vi "B-Field Control Signal Generator.vi"() -> ()   [LabVIEW 2009]
doc: "I. Description:\nThis example demonstrates how to continuously output a waveform using an internal sample clock and a digital start trigger.\n\nII. Instructions for Running:\n1. Select the Physical Channel to correspond to where your signal is output on the DAQ device.\n2. Enter the Minimum and Maximum Voltage Ranges.\n3. Specify the Desired Frequency of the output Waveform\n4. Select the Digital Trigger Source.\n5. Specify the desired Trigger Edge.\n6. Enter the Waveform Information. See the documentation of the Waveform Buffer Generation SubVI for information on each parameter.\n\nIII. Block Diagram Steps:\n1. Create an Analog Output Voltage Task\n2.Call the DAQmx Timing (Use Waveform) VI which sets the sample clock rate based on the input waveform parameters, and set the sample mode to Continuous.\n3. Define the Triggering parameters: Source and Edge\n4. Write the waveform to the output buffer.\n5. Call the Start VI.\n6. Loop continuously until the user presses the Stop button. Check for errors every 100 ms using the Is Task Done? VI\n7. Call the Clear Task VI to clear the Task.\n8. Use the popup dialog box to display an error or warning if any.\n\nIV. I/O Connections Overview:\nMake sure your signal output terminal matches the Physical Channel I/O Control. Also, make sure your digital trigger terminal matches the Trigger Source Control. For further connection information, refer to your hardware reference manual."
uses:
  B-Generator States.ctl
  <vilib>/Utility/error.llb/DialogType.ctl
  <vilib>/DAQmx/write.llb/DAQmx Write (Analog 1D DBL 1Chan NSamp).vi
  <vilib>/DAQmx/configure/trigger.llb/DAQmx Start Trigger (Digital Edge).vi
  <vilib>/DAQmx/configure/timing.llb/DAQmx Timing (Sample Clock).vi
  <vilib>/DAQmx/create/channels.llb/DAQmx Create Channel (AO-Voltage-Basic).vi
  Program Files (x86)/National Instruments/LabVIEW 2009/resource/objmgr/daqmx.rc
panel:
  in  "V5":dbl[unit]=4.0
  in  "V4":dbl[unit]=1.0
  in  "V3":dbl[unit]=-3.0
  in  "V2":dbl[unit]=-5.0
  in  "V1":dbl[unit]=5.0
  in  "D":dbl[unit]=9.999999999999999e-05
  in  "C":dbl[unit]=9.999999999999999e-05
  in  "B":dbl[unit]=9.999999999999999e-05
  in  "A":dbl[unit]=9.999999999999999e-05
  out "B-Field Control Signal":dbl[](graph)
  in  "stop":bool
  # "Example Diagram"
  # "Voltages"
  # "Interval Times"
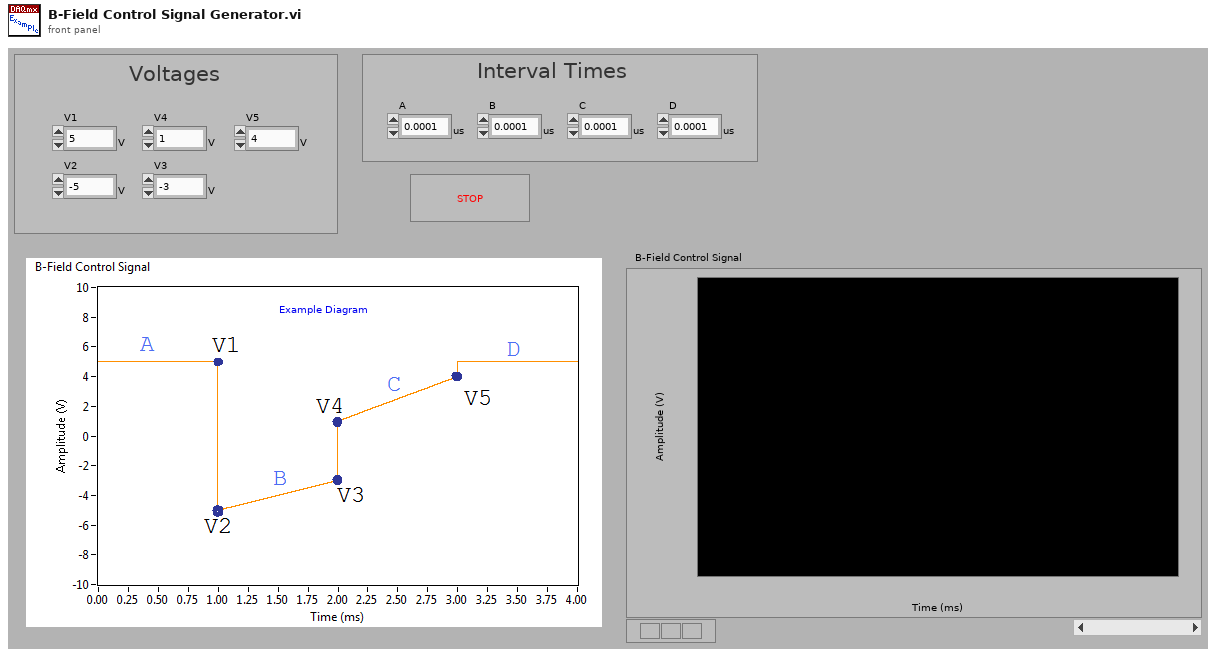
[diagram p1: front panel]
types:
  T1 = typedef "DialogType.ctl" = u16
  T2 = typedef "B-Generator States.ctl" = enum16{"Initialize", "Start Task", "Check Task", "Stop Task", "Stop"}
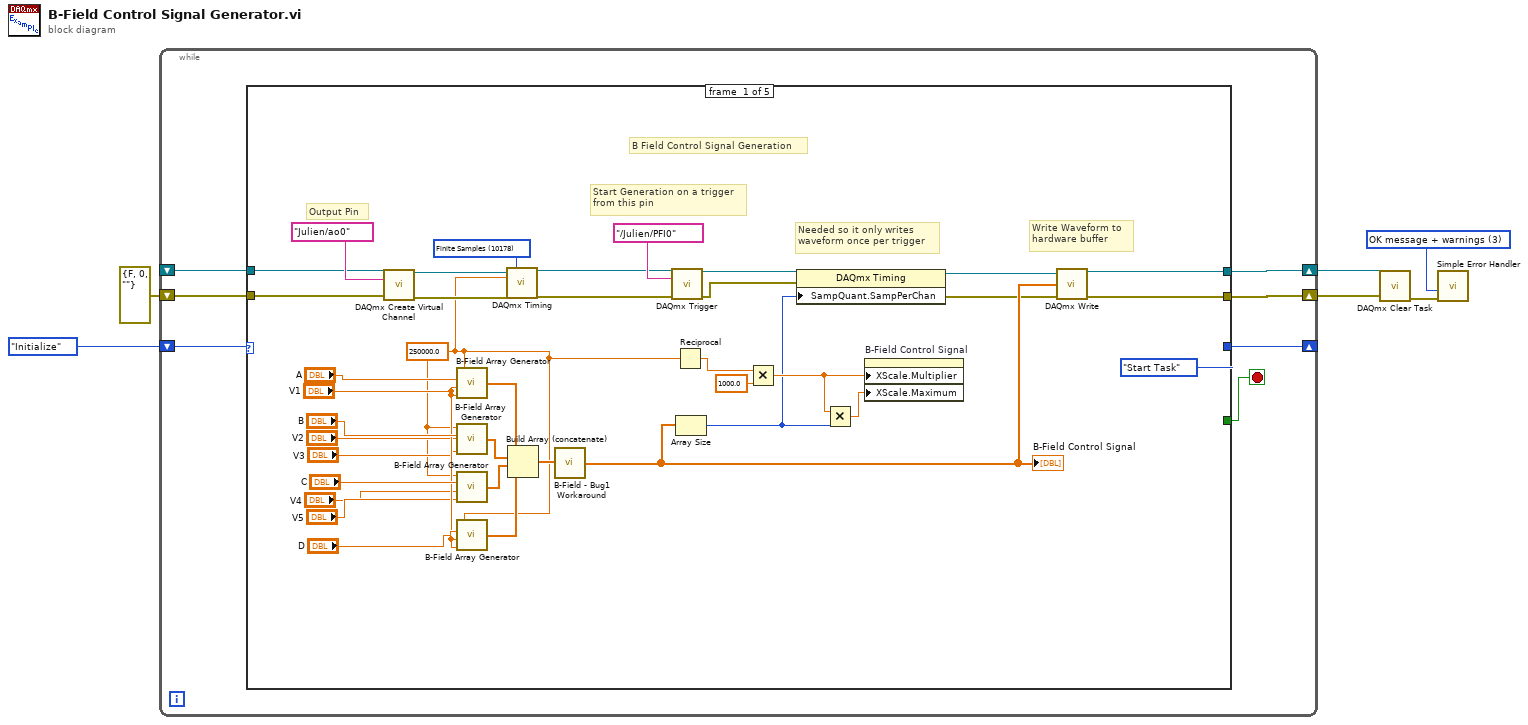
[diagram p0: block diagram]
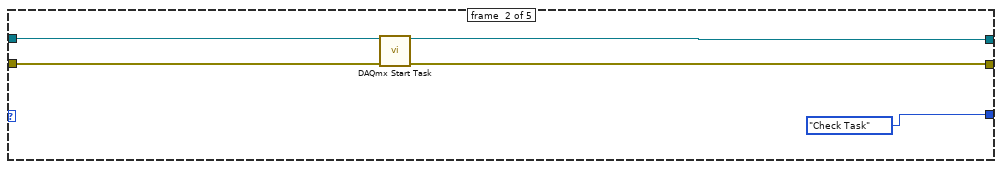
[diagram p2: hidden frame]
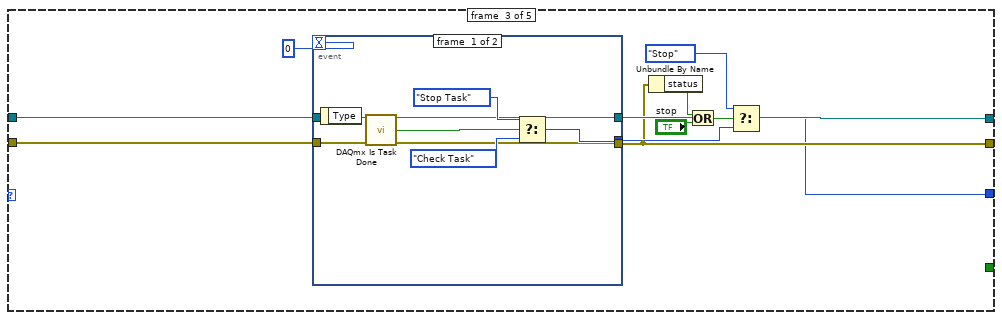
[diagram p3: hidden frame]
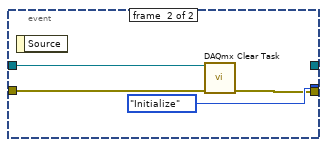
[diagram p4: hidden frame]
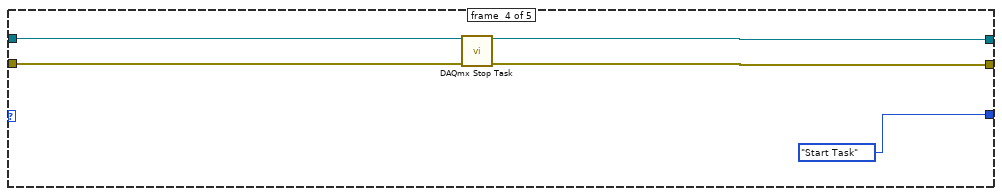
[diagram p5: hidden frame]
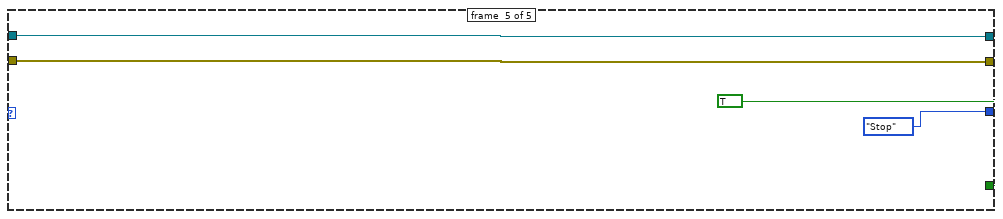
[diagram p6: hidden frame]
diagram:
  w6 = T1 3 items=["no dialog", "OK message", "continue or stop message", "OK message + warnings", "continue/stop + warnings"] ("type of dialog (OK msg:1)")
  n1 = while {
    shift-right: [w10] -> _
    shift-left: B-Generator_States."Initialize" ("B-Generator States") -> [w11]
    shift-right: [w12] -> w3
    shift-left: errorcluster {"status"=FALSE, "code"=0, "source"=""} ("error out") -> [w7]
    shift-right: [w13] -> w4
    shift-left: _ -> [w8]
    stop <- w9 stop-if-true
    n2 = case shown="\"Initialize\"" w11 {
      tunnel: [w29 w52 w58 w81 w85] -> w13
      tunnel: [w28 w53 w57 w80 w84] -> w12
      tunnel: [B-Generator_States."Start Task" ("B-Generator States") B-Generator_States."Check Task" ("B-Generator States") w56 B-Generator_States."Start Task" ("B-Generator States") B-Generator_States."Stop" ("B-Generator States")] -> w10
      tunnel: [_ _ _ _ TRUE] -> w9
      tunnel: w8 -> [w27 w55 w60 w83 w85]
      tunnel: w7 -> [w34 w54 w59 w82 w84]
      frame #0 {
        w23 = 250000.0
        w41 = 10178 items=["Finite Samples"=10178, "Continuous Samples"=10123] ("sample mode")
        # "B Field Control Signal Generation"
        # "Write Waveform to\nhardware buffer"
        # "Output Pin"
        # "Start Generation on a trigger \nfrom this pin"
        # "Needed so it only writes \nwaveform once per trigger"
        n3 = call-poly <vilib>:"DAQmx Create Virtual Channel.vi"("task in"=w27, "physical channels"=tag "Julien/ao0" ("Physical Channels"), "error in"=w34) -> ("task out"=w36:refnum<k21>, "error out"=w35:errorcluster)  [unwired: 7 in, 4 out]
        n4 = call "B-Field Array Generator.vi"("Final Voltage"="V1", "Initial Voltage"="V1", "Time"="A", "Sample Rate"=w23) -> ("Voltage Ouputs"=w33:dbl[])
        n5 = call "B-Field Array Generator.vi"("Final Voltage"="V3", "Initial Voltage"="V2", "Time"="B", "Sample Rate"=w23) -> ("Voltage Ouputs"=w30:dbl[])
        n6 = call "B-Field Array Generator.vi"("Final Voltage"="V5", "Initial Voltage"="V4", "Time"="C", "Sample Rate"=w23) -> ("Voltage Ouputs"=w31:dbl[])
        n7 = call "B-Field Array Generator.vi"("Final Voltage"="V1", "Initial Voltage"="V1", "Time"="D", "Sample Rate"=w23) -> ("Voltage Ouputs"=w32:dbl[])
        n8 = call-poly <vilib>:"DAQmx Timing.vi"("task/channels in"=w36, "sample mode"=w41, "rate"=w23, "error in"=w35) -> ("task out"=w19:refnum<k21>, "error out"=w39:errorcluster)  [unwired: 3 in, 7 out]
        n9 = Build Array (concatenate)(w33, w30, w31, w32) -> (w26:dbl[])
        n10 = call "B-Field - Bug1 Workaround.vi"("Array 2"=w26) -> ("Array"=w24:dbl[])
        "B-Field Control Signal" <- w24
        n11 = call-poly <vilib>:"DAQmx Trigger.vi"("task/channels in"=w19, "source"=tag "/Julien/PFI0" ("Trigger Source"), "error in"=w39) -> ("task out"=w18:refnum<k21>, "error out"=w17:errorcluster)  [unwired: 1 in, 10 out]
        n12 = Reciprocal(x=w23) -> (1/x=w22:dbl)
        n13 = Array Size(array=w24) -> (size(s)=w14:i32)
        n14 = Multiply(x=w22, y=1000.0) -> (x*y=w21:dbl)
        n15 = property class="DAQmx Timing"(reference=w18, error in=w17, "SampQuant.SampPerChan"=w14) -> (reference out=w16:refnum<k21>, error out=w15:errorcluster)
        n16 = Multiply(x=w21, y=w14) -> (x*y=w20:dbl)
        n17 = property on="B-Field Control Signal" class="WFGraph (strict)"("XScale.Multiplier"=w21, "XScale.Maximum"=w20) -> ()  [unwired: 2 in, 2 out]
        n18 = call-poly <vilib>:"DAQmx Write.vi"("task/channels in"=w16, "data"=w24, "error in"=w15) -> ("task out"=w29:refnum<k21>, "error out"=w28:errorcluster)  [unwired: 1 in, 10 out]
      }
      frame #1 {
        n19 = call <vilib>:"DAQmx Start Task.vi"("task/channels in"=w55, "error in"=w54) -> ("task out"=w52:refnum<k21>, "error out"=w53:errorcluster)  [unwired: 12 out]
      }
      frame #2 {
        n20 = event shown="[1] \"A\", \"B\", \"C\", \"D\", \"V1\", \"V2\", \"V3\", \"V4\", \"V5\": Value Change" {
          selector: _ -> [_ _]
          dyn-events: _ -> [_ _]
          timeout: 0 -> [_ _]
          tunnel: [w69 B-Generator_States."Initialize" ("B-Generator States")] -> w61
          tunnel: [w67 _] -> w58
          tunnel: w60 -> [w74 w77]
          tunnel: w59 -> [w73 w76]
          tunnel: [w68 w75] -> w57
          event #0 {
            n21 = event-data() -> ()  [unwired: 2 out]
            n22 = call <vilib>:"DAQmx Is Task Done.vi"("task/channels in"=w74, "error in"=w73) -> ("task out"=w67:refnum<k21>, "task done?"=w72:bool, "error out"=w68:errorcluster)  [unwired: 1 in, 10 out]
            n23 = Select(t=B-Generator_States."Stop Task" ("B-Generator States"), s=w72, f=B-Generator_States."Check Task" ("B-Generator States")) -> (s? t:f=w69:T2)
          }
          event #1 {
            n24 = event-data() -> ()  [unwired: 2 out]
            n25 = call <vilib>:"DAQmx Clear Task.vi"("task in"=w77, "error in"=w76) -> ("error out"=w75:errorcluster)  [unwired: 13 out]
          }
        }
        n26 = Unbundle By Name(w57) -> ("status"=w65:bool)
        n27 = Or(x=w65, y="stop") -> (x .or. y?=w64:bool)
        n28 = Select(t=B-Generator_States."Stop" ("B-Generator States"), s=w64, f=w61) -> (s? t:f=w56:T2)
      }
      frame #3 {
        n29 = call <vilib>:"DAQmx Stop Task.vi"("task/channels in"=w83, "error in"=w82) -> ("task out"=w81:refnum<k21>, "error out"=w80:errorcluster)  [unwired: 12 out]
      }
      frame #4 {
      }
    }
  }
  n30 = call <vilib>:"DAQmx Clear Task.vi"("task in"=w4, "error in"=w3) -> ("error out"=w5:errorcluster)  [unwired: 13 out]
  n31 = call <vilib>:"Simple Error Handler.vi"("type of dialog (OK msg:1)"=w6, "error in (no error)"=w5) -> ()  [unwired: 8 out]
